vi "translate.vi"(8 "error in (no error)":errorcluster, 10 "vector":dbl[](array[numeric]), 11 "PointCollection in":refnum<class "PointCollection.lvclass">) -> (0 "error out":errorcluster, 3 "PointCollection out":refnum<class "PointCollection.lvclass">)   [LabVIEW 2010, in "PointCollection.lvclass"]
uses:
  PointCollection.lvclass
  PointCollection.lvclass/PointCollection.ctl
  mode_enum.ctl
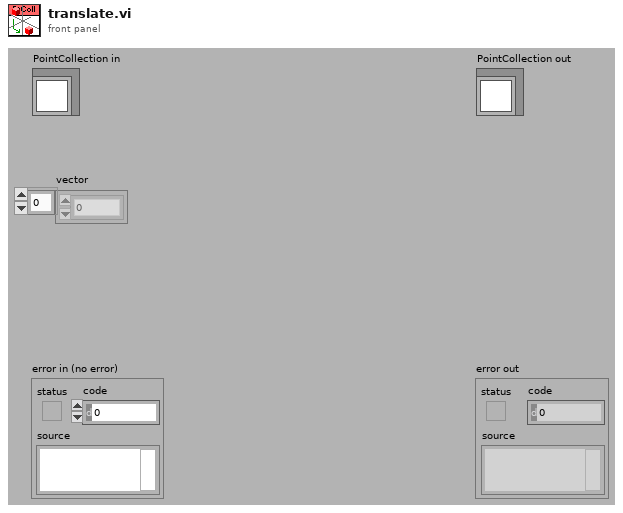
[diagram p1: front panel]
types:
  T1 = typedef "PointCollection.lvclass/mode_enum.ctl" = enum16{"points first", "dimensions first"}
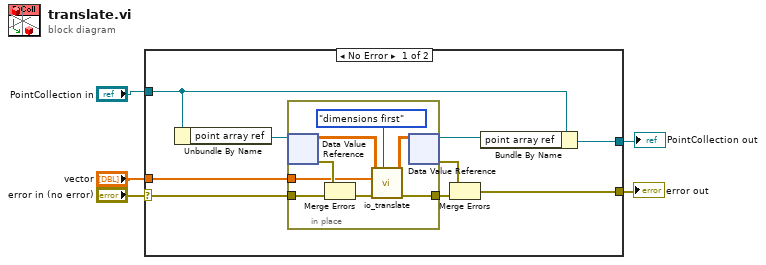
[diagram p0: block diagram]
diagram:
  n1 = case shown="No Error" "error in (no error)" {
    selector: "error in (no error)" -> [w14 w24]
    tunnel: [w7 w24] -> w4
    tunnel: [w9 w23] -> w2
    tunnel: "PointCollection in" -> [w10 w23]
    tunnel: "vector" -> [w13 _]
    frame No Error {
      n2 = Unbundle By Name(w10) -> ("point array ref"=w12:refnum<data-value>)
      n3 = in-place {
        in-place-border: w14 -> [w20]
        in-place-border: [w22] -> w6
        in-place-border: w13 -> [w18]
        n4 = in-place-dvr #1(w12) -> (w17:dbl[][], w21:errorcluster)
        n5 = Merge Errors(w21, w20) -> (w19:errorcluster)
        n6 = call "io_translate.vi"("mode"=mode_enum."dimensions first", "error in (no error)"=w19, "vector"=w18, "points in"=w17) -> ("error out"=w22:errorcluster, "points out"=w16:dbl[][])  [unwired: 6 in]
        n7 = in-place-dvr #1(w16) -> (w11:refnum<data-value>, w8:errorcluster)
      }
      n8 = Merge Errors(w8, w6) -> (w7:errorcluster)
      n9 = Bundle By Name(cluster=w10, "point array ref"=w11) -> (w9:refnum<class "PointCollection.lvclass">)
    }
    frame Error {
    }
  }
  "error out" <- w4
  "PointCollection out" <- w2
